vi "Read PubDataEvents.vi"(11 "UserEvents in":refnum<class "UserEvents.lvclass">) -> (2 "PubDataEvents":T1, 3 "UserEvents out":refnum<class "UserEvents.lvclass">)   [LabVIEW 2015, in "UserEvents.lvclass"]
uses:
  UserEvents.lvclass
  Typedefs/PubDataEvents.ctl
  Typedefs/StateSelector.ctl
  Typedefs/OutputData.ctl
  Typedefs/InputData.ctl
  Typedefs/ForceDemand.ctl
  <userlib>/Common/Devices/DistanceGauge/Typedefs/Distance Data.ctl
  Typedefs/ControllerData.ctl
  Typedefs/TestStatus.ctl
  Typedefs/StiffnessData.ctl
  UserEvents.lvclass/UserEvents.ctl
  Typedefs/M1M3SSSTypedefs.lvlib
  <userlib>/Common/Devices/DistanceGauge/DistanceGauge.lvlib
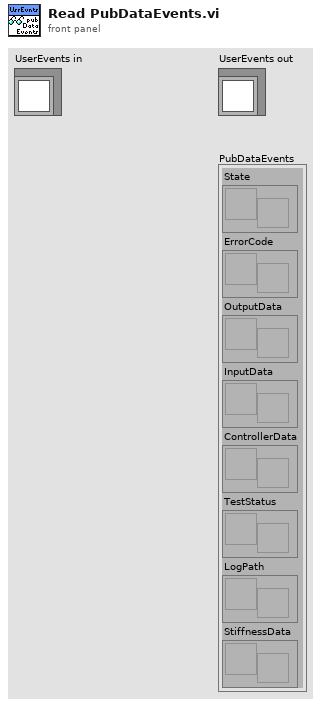
[diagram p1: front panel]
types:
  T1 = typedef "M1M3SSSTypedefs.lvlib/PubDataEvents.ctl" = cluster{"State":refnum<user-event>, "ErrorCode":refnum<user-event>, "OutputData":refnum<user-event>, "InputData":refnum<user-event>, "ControllerData":refnum<user-event>, "TestStatus":refnum<user-event>, "LogPath":refnum<user-event>, "StiffnessData":refnum<user-event>}
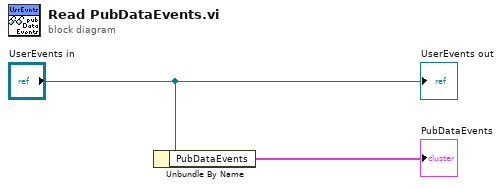
[diagram p0: block diagram]
diagram:
  n1 = Unbundle By Name("UserEvents in") -> ("PubDataEvents"=→"PubDataEvents":T1)
  "UserEvents out" <- "UserEvents in"
